vi "GlobalVariables.vi"() -> ()   [LabVIEW 2020, in "AIM MIL-STD-1553 Scripting.lvlib"]
uses:
  AIM MIL-STD-1553 Scripting.lvlib
panel:
  in  "g_IncludeDirectionSection":bool
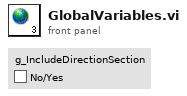
[diagram p1: front panel]
diagram:
